vi "Depth Image Continuous Acquisition.vi"() -> ()   [LabVIEW 2011]
uses:
  <vilib>/LabVIEW Hacker/LVH-Interface-for-Kinect/LVH-Interface-for-Kinect.lvlib
panel:
  out "Kinect Depth Image":T1(plugin-control)
  out "Frame Number":i32
  in  "Stop Button":bool
  # "This example continuously acquires the depth image from the Kinect ."
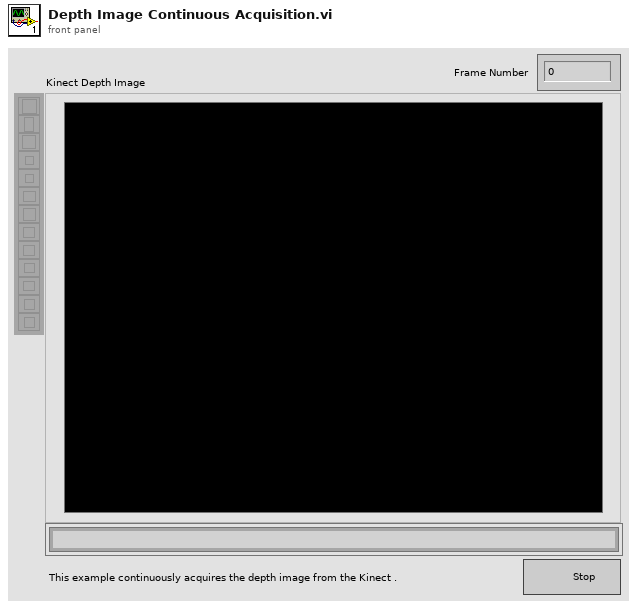
[diagram p1: front panel]
types:
  T1 = typedef "IMAQ Image.ctl" = refnum<image>
  T2 = typedef "Image Type" = u32
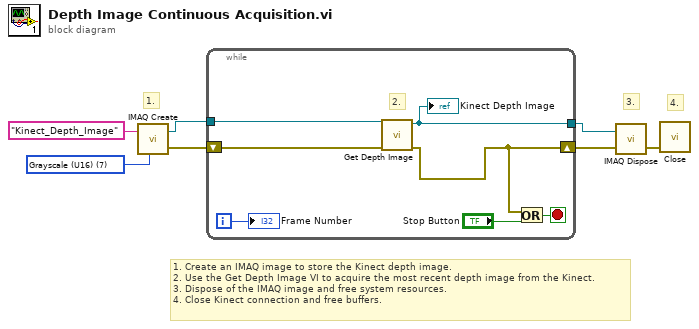
[diagram p0: block diagram]
diagram:
  w3 = T2 7 items=["Grayscale (U8)", "Grayscale (I16)", "Grayscale (SGL)", "Complex (CSG)", "RGB (U32)", "HSL (U32)", "RGB (U64)", "Grayscale (U16)"] ("Image Type")
  # "4."
  # "1. Create an IMAQ image to store the Kinect depth image.\n2. Use the Get Depth Image VI to acquire the most recent depth image from the Kinect.\n3. Dispose of the IMAQ image and free system resources.\n4. Close Kinect connection and free buffers."
  # "3."
  # "1."
  n1 = call "IMAQ Create"("Image Name"="Kinect_Depth_Image", "Image Type"=w3) -> ("New Image"=w7:T1, "error out"=w5:errorcluster)  [unwired: 3 in]
  n2 = while {
    tunnel: w7 -> [w13]
    tunnel: [w9] -> w6
    shift-right: [w8] -> w2
    shift-left: w5 -> [w10]
    i -> [w14]
    stop <- w11 stop-if-true
    # "2."
    n3 = call <vilib>:"Get Depth Image.vi"("Error In"=w10, "Image"=w13) -> ("Error Out"=w8:errorcluster, "Image Out"=w9:T1)  [unwired: 7 in, 1 out]
    "Kinect Depth Image" <- w9
    n4 = Or(x=w8, y="Stop Button") -> (x .or. y?=w11:bool)
    "Frame Number" <- w14
  }
  n5 = call "IMAQ Dispose"("Image"=w6, "error in (no error)"=w2) -> ("error out"=w1:errorcluster)  [unwired: 4 in]
  n6 = call <vilib>:"Close.vi"("Error In"=w1) -> ()  [unwired: 10 in, 1 out]
